vi "Test Arena.vi"() -> ()   [LabVIEW 2013]
panel:
  out "XY Graph":cluster{"Y":dbl[], "Y":dbl[]}[](graph)
  in  "Start Coordinate (mm)":dbl
  in  "Target Coordinate (mm)":dbl min=0.0
  in  "Creep (mm)":dbl
  out "Selected Speed Control Case":T1(ring)
  in  "Overrun (mm)":dbl
  in  "stop":bool
  in  "Decel Rate (mm/s^2) 2":dbl
  in  "Accel Rate (mm/s^2)":dbl
  in  "Vmax (mm/s)":dbl
  in  "Timestep (dt)":dbl
  in  "Vcreep (mm/s)":dbl
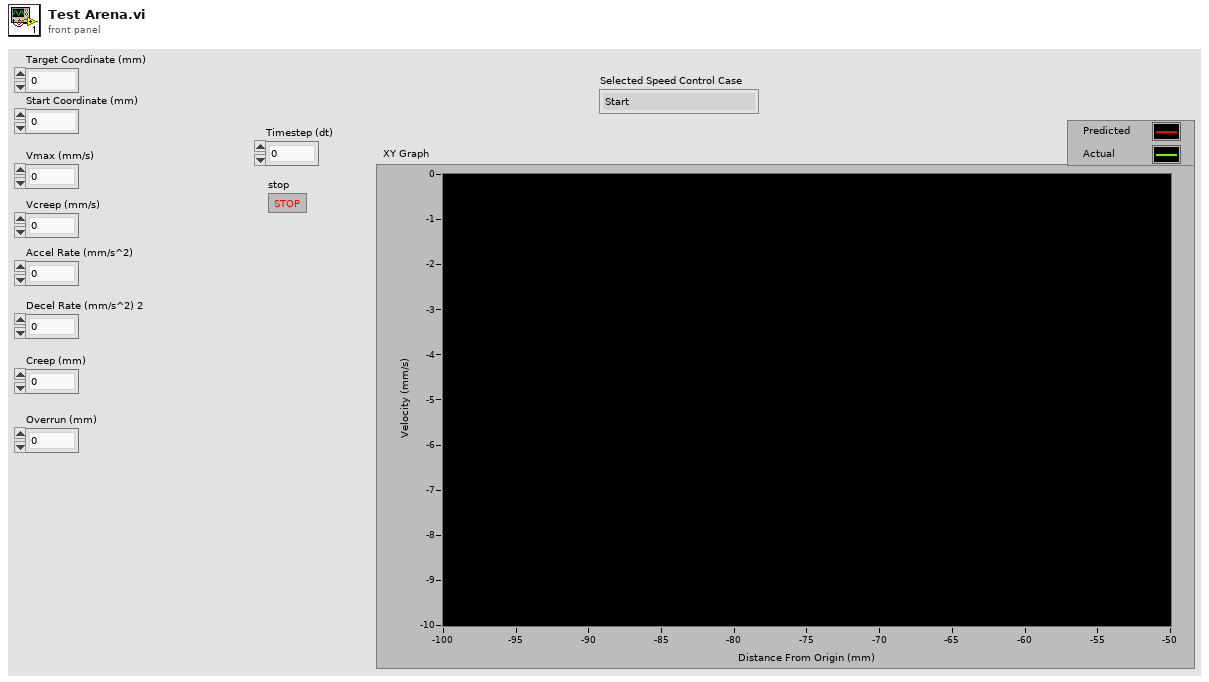
[diagram p1: front panel]
types:
  T1 = enum16{"Start", "Accelerate", "Hold Vmax", "Decelerate", "Hold at Vcreep", "Stop"}
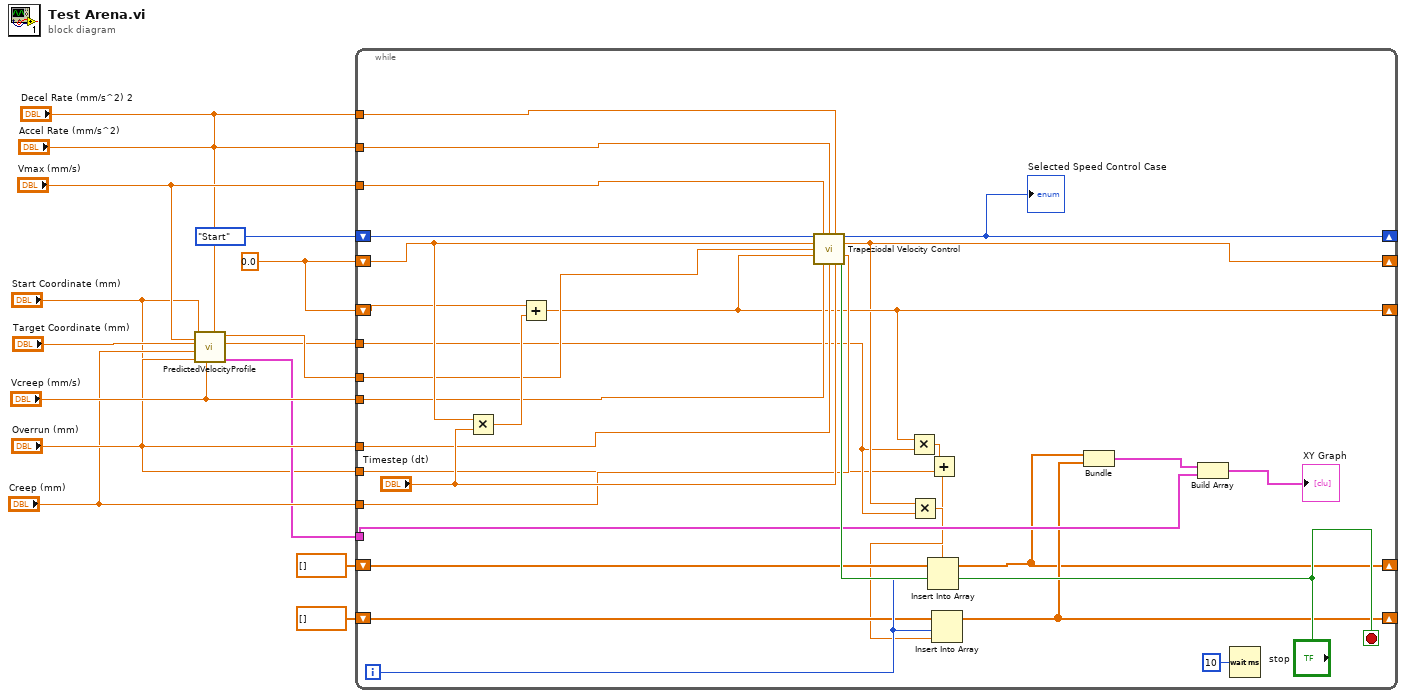
[diagram p0: block diagram]
diagram:
  w2 = 0.0 ("Speed Command (mm/s)")
  n1 = call "PredictedVelocityProfile.vi"("Decel_mm/s^2"="Decel Rate (mm/s^2) 2", "Accel_mm/s^2"="Accel Rate (mm/s^2)", "V_Creep_mm/s"="Vcreep (mm/s)", "V_Max_mm/s"="Vmax (mm/s)", "S_Overrun_mm"="Overrun (mm)", "S_Creep_mm"="Creep (mm)", "Target Coordinate (mm)"="Target Coordinate (mm)", "Start Coordinate (mm)"="Start Coordinate (mm)") -> ("PredictedVelocityProfile"=w6:cluster{dbl[], cdb[]}, "Direction Request"=w3:dbl, "Absolute Distance to Move (mm)"=w14:dbl)  [unwired: 1 in]
  n2 = while {
    shift-right: [w40] -> _
    shift-left: T1."Start" ("Selected Speed Control Case") -> [w45]
    shift-right: [w20] -> _
    shift-left: w2 -> [w44]
    shift-right: [w22] -> _
    shift-left: w2 -> [w23]
    tunnel: "Decel Rate (mm/s^2) 2" -> [w38]
    tunnel: "Accel Rate (mm/s^2)" -> [w37]
    tunnel: "Vmax (mm/s)" -> [w36]
    tunnel: w14 -> [w35]
    tunnel: "Creep (mm)" -> [w34]
    tunnel: "Overrun (mm)" -> [w33]
    tunnel: "Vcreep (mm/s)" -> [w32]
    tunnel: w3 -> [w18]
    shift-right: [w24] -> _
    shift-left: dbl[] [] -> [w30]
    shift-right: [w25] -> _
    shift-left: dbl[] [] -> [w29]
    tunnel: w6 -> [w27]
    tunnel: "Start Coordinate (mm)" -> [w16]
    i -> [w31]
    stop <- "stop" stop-if-true
    n3 = Multiply(x=w44, y="Timestep (dt)") -> (x*y=w43:dbl)
    n4 = Add(x=w23, y=w43) -> (x+y=w22:dbl)
    n5 = call "Trapeziodal Velocity Control.vi"("Active Speed Control Case"=w45, "Vmax (mm/s)"=w36, "Accel Rate (mm/s^2)"=w37, "Decel Rate (mm/s^2) 2"=w38, "Current Speed (mm/s)"=w44, "Target Distance (mm)"=w35, "Actual Distance (mm)"=w22, "Creep  Distance (mm)"=w34, "Vcreep (mm/s)"=w32, "Overrun Distance (mm)"=w33, "Timestep (dt)"="Timestep (dt)", "stop or error"="stop") -> ("Selected Speed Control Case"=w40:T1, "Speed Command (mm/s)"=w20:dbl)  [unwired: 2 in]
    "Selected Speed Control Case" <- w40
    n6 = Multiply(x=w22, y=w18) -> (x*y=w21:dbl)
    n7 = Multiply(x=w20, y=w18) -> (x*y=w19:dbl)
    n8 = Add(x=w21, y=w16) -> (x+y=w17:dbl)
    n9 = Insert Into Array(array=w30, index=w31, new element=w17) -> (w24:dbl[])
    n10 = Insert Into Array(array=w29, index=w31, new element=w19) -> (w25:dbl[])
    n11 = Bundle(w24, w25) -> (w26:cluster{dbl[], dbl[]})  [unwired: 1 in]
    n12 = Build Array(w26, w27) -> (→"XY Graph":cluster{dbl[], cdb[]}[])
    n13 = Wait (ms)(milliseconds to wait=u32 10) -> ()  [unwired: 1 out]
  }
